vi "Show Hide Controls.vi"(8 "error in (no error)":errorcluster, 10 "Hidable Controls":T1, 11 "TDMS datalogger configuration":refnum<class "TDMS datalogger configuration.lvclass">) -> (0 "error out":errorcluster, 3 "Datalogger configuration out":refnum<class "TDMS datalogger configuration.lvclass">)   [LabVIEW 2015, in "TDMS datalogger editor node.lvclass"]
uses:
  TDMS datalogger editor node.lvclass
  module/configuration/TDMS datalogger configuration.lvclass
  module/configuration/Hidable controls.ctl
  module/configuration/TDMS datalogger configuration.lvclass/TDMS datalogger configuration.ctl
  module/configuration/Read add enable channel.vi
  module/configuration/Read Logging Type.vi
  module/configuration/Read Trigger Type.vi
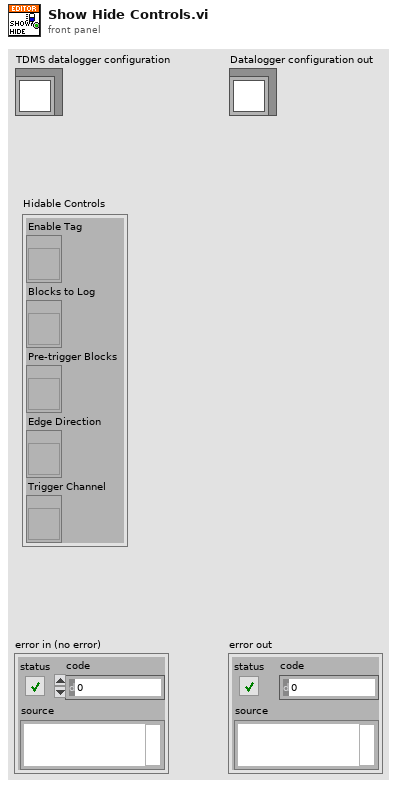
[diagram p1: front panel]
types:
  T1 = typedef "TDMS datalogger editor node.lvclass/Hidable controls.ctl" = cluster{"Enable Tag":refnum<vi>, "Blocks to Log":refnum<vi>, "Pre-trigger Blocks":refnum<vi>, "Edge Direction":refnum<vi>, "Trigger Channel":refnum<vi>}
  T2 = typedef "TDMS datalogger configuration.lvclass/Logging Type.ctl" = enum16{"Continuous", "Finite"}
  T3 = typedef "TDMS datalogger configuration.lvclass/Trigger Type.ctl" = enum16{"None", "Start"}
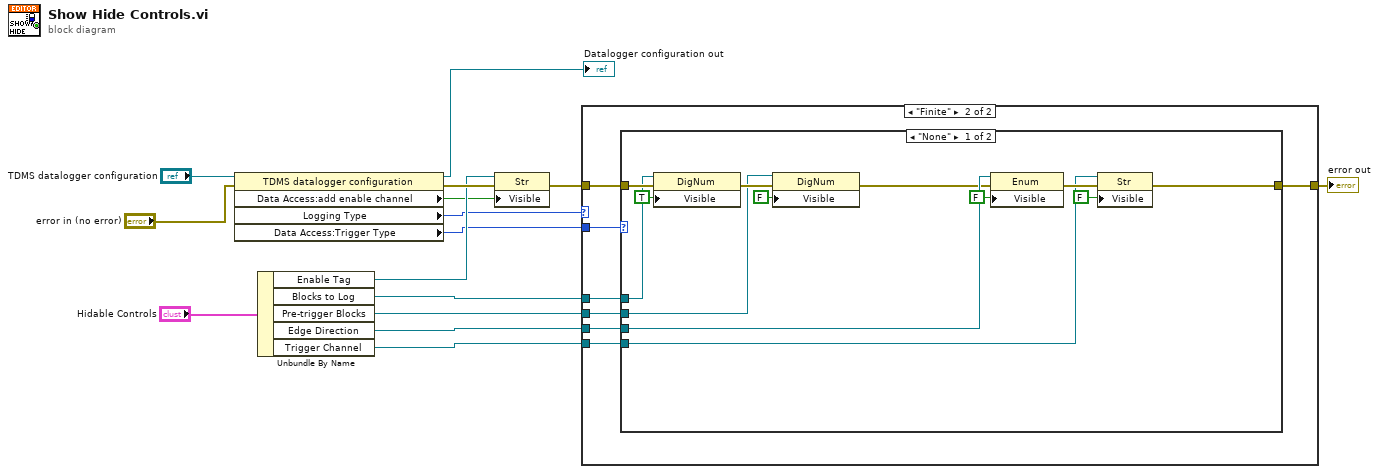
[diagram p0: block diagram]
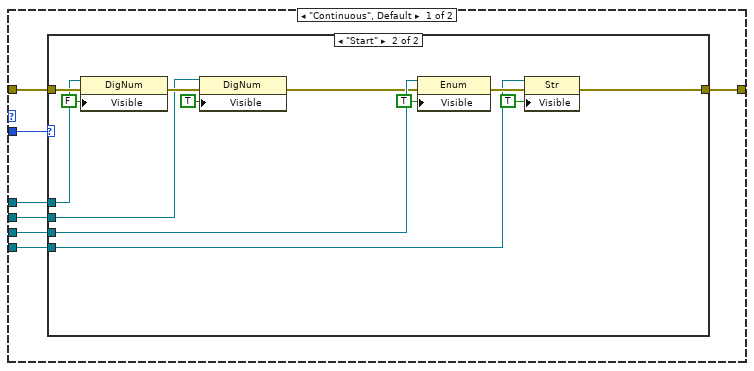
[diagram p2: hidden frame]
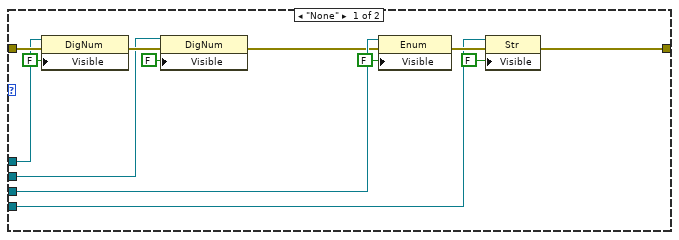
[diagram p3: hidden frame]
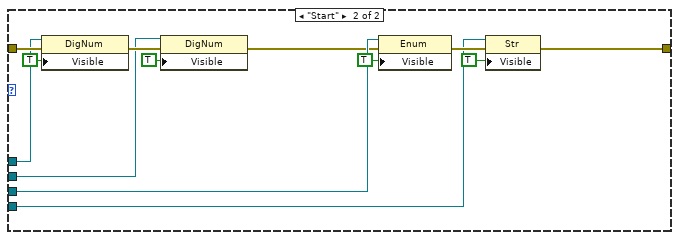
[diagram p4: hidden frame]
diagram:
  n1 = property class="TDMS datalogger configuration"(reference="TDMS datalogger configuration", error in="error in (no error)") -> (reference out=→"Datalogger configuration out":refnum<class "TDMS datalogger configuration.lvclass">, error out=w13:errorcluster, "Data Access:add enable channel"=w11:bool, "Logging Type"=w10:T2, "Data Access:Trigger Type"=w9:T3)
  n2 = Unbundle By Name("Hidable Controls") -> ("Enable Tag"=w12:refnum<vi>, "Blocks to Log"=w8:refnum<vi>, "Pre-trigger Blocks"=w6:refnum<vi>, "Edge Direction"=w5:refnum<vi>, "Trigger Channel"=w4:refnum<vi>)
  n3 = property class="Str"(reference=w12, error in=w13, "Visible"=w11) -> (error out=w7:errorcluster)  [unwired: 1 out]
  n4 = case shown="\"Finite\"" w10 {
    tunnel: w9 -> [w22 w55]
    tunnel: w8 -> [w21 w54]
    tunnel: w7 -> [w20 w53]
    tunnel: w6 -> [w19 w52]
    tunnel: w5 -> [w18 w51]
    tunnel: w4 -> [w17 w50]
    tunnel: [w16 w49] -> w2
    frame "Continuous", Default {
      n5 = case shown="\"Start\"" w22 {
        tunnel: w21 -> [w34 w47]
        tunnel: w20 -> [w35 w48]
        tunnel: w19 -> [w32 w45]
        tunnel: w18 -> [w29 w42]
        tunnel: w17 -> [w26 w39]
        tunnel: [w24 w36] -> w16
        frame "None" {
          n6 = property class="DigNum"(reference=w34, error in=w35, "Visible"=FALSE) -> (error out=w33:errorcluster)  [unwired: 1 out]
          n7 = property class="DigNum"(reference=w32, error in=w33, "Visible"=FALSE) -> (error out=w23:errorcluster)  [unwired: 1 out]
          n8 = property class="Enum"(reference=w29, error in=w23, "Visible"=FALSE) -> (error out=w27:errorcluster)  [unwired: 1 out]
          n9 = property class="Str"(reference=w26, error in=w27, "Visible"=FALSE) -> (error out=w24:errorcluster)  [unwired: 1 out]
        }
        frame "Start" {
          n10 = property class="DigNum"(reference=w47, error in=w48, "Visible"=FALSE) -> (error out=w46:errorcluster)  [unwired: 1 out]
          n11 = property class="DigNum"(reference=w45, error in=w46, "Visible"=TRUE) -> (error out=w37:errorcluster)  [unwired: 1 out]
          n12 = property class="Enum"(reference=w42, error in=w37, "Visible"=TRUE) -> (error out=w40:errorcluster)  [unwired: 1 out]
          n13 = property class="Str"(reference=w39, error in=w40, "Visible"=TRUE) -> (error out=w36:errorcluster)  [unwired: 1 out]
        }
      }
    }
    frame "Finite" {
      n14 = case shown="\"None\"" w55 {
        tunnel: w54 -> [w67 w80]
        tunnel: w53 -> [w68 w81]
        tunnel: w52 -> [w65 w78]
        tunnel: w51 -> [w62 w75]
        tunnel: w50 -> [w59 w72]
        tunnel: [w57 w69] -> w49
        frame "None" {
          n15 = property class="DigNum"(reference=w67, error in=w68, "Visible"=TRUE) -> (error out=w66:errorcluster)  [unwired: 1 out]
          n16 = property class="DigNum"(reference=w65, error in=w66, "Visible"=FALSE) -> (error out=w56:errorcluster)  [unwired: 1 out]
          n17 = property class="Enum"(reference=w62, error in=w56, "Visible"=FALSE) -> (error out=w60:errorcluster)  [unwired: 1 out]
          n18 = property class="Str"(reference=w59, error in=w60, "Visible"=FALSE) -> (error out=w57:errorcluster)  [unwired: 1 out]
        }
        frame "Start" {
          n19 = property class="DigNum"(reference=w80, error in=w81, "Visible"=TRUE) -> (error out=w79:errorcluster)  [unwired: 1 out]
          n20 = property class="DigNum"(reference=w78, error in=w79, "Visible"=TRUE) -> (error out=w70:errorcluster)  [unwired: 1 out]
          n21 = property class="Enum"(reference=w75, error in=w70, "Visible"=TRUE) -> (error out=w73:errorcluster)  [unwired: 1 out]
          n22 = property class="Str"(reference=w72, error in=w73, "Visible"=TRUE) -> (error out=w69:errorcluster)  [unwired: 1 out]
        }
      }
    }
  }
  "error out" <- w2
